vi "单路通断器（DBL).vi"(1 "默认值":dbl=nan, 2 "直通？":bool=TRUE, 3 "X_In":dbl=100.0) -> (0 "X_Out":dbl)   [LabVIEW 2012]
doc: "功能：\n\n返回一个枚举，表明输入数的范围，用于三段比较。\n\n\nCSXCS_366创建。"
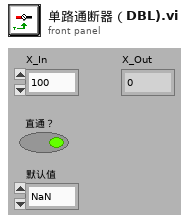
[diagram p1: front panel]
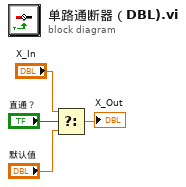
[diagram p0: block diagram]
diagram:
  n1 = Select(t="X_In", s="直通？", f="默认值") -> (s? t:f=→"X_Out":dbl)
